vi "exit_loops.vi"(8 "error in (no error)":errorcluster, 11 "Message Queues in":T1) -> (0 "error out":errorcluster)   [LabVIEW 2015]
uses:
  support/Message Queue/All Message Queues.ctl
  support/Message Queue/Message Cluster.ctl
  support/Message Queue/Enqueue Message (Single).vi
  support/Message Queue/regser Message Queue.lvlib
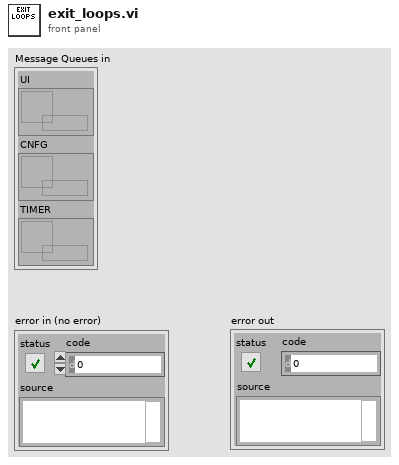
[diagram p1: front panel]
types:
  T1 = typedef "regser Message Queue.lvlib/All Message Queues.ctl" = cluster{"UI":refnum<queue>, "CNFG":refnum<queue>, "TIMER":refnum<queue>}
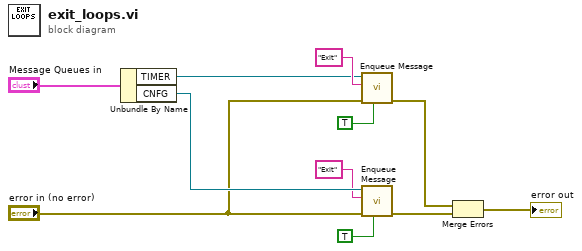
[diagram p0: block diagram]
diagram:
  n1 = Unbundle By Name("Message Queues in") -> ("TIMER"=w1:refnum<queue>, "CNFG"=w5:refnum<queue>)
  n2 = call-poly "Enqueue Message.vi"("Priority Message? (F)"=TRUE, "error in (no error)"="error in (no error)", "Message"="Exit", "Message Queue"=w1) -> ("error out"=w6:errorcluster)  [unwired: 6 in, 1 out]
  n3 = call-poly "Enqueue Message.vi"("Priority Message? (F)"=TRUE, "error in (no error)"="error in (no error)", "Message"="Exit", "Message Queue"=w5) -> ("error out"=w9:errorcluster)  [unwired: 6 in, 1 out]
  n4 = Merge Errors(w6, w9) -> (→"error out":errorcluster)
